vi "Load plugin from enum.vi"(4 "error in (no error)":errorcluster, 7 "Plugin type":T1) -> (0 "error out":errorcluster, 3 "Generic Plugin out":refnum<class "Generic Plugin.lvclass">)   [LabVIEW 2020, in "Generic Plugin.lvclass"]
uses:
  Generic Plugin.lvclass
  Plugin Type.ctl
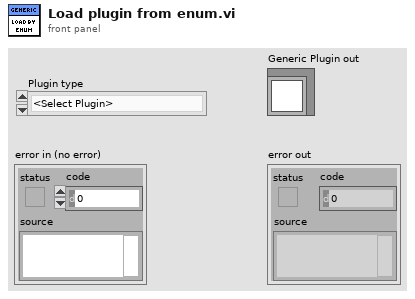
[diagram p1: front panel]
types:
  T1 = typedef "Generic Plugin.lvclass/Plugin Type.ctl" = enum16{"<Select Plugin>", "Orange", "Blue", "Red"}
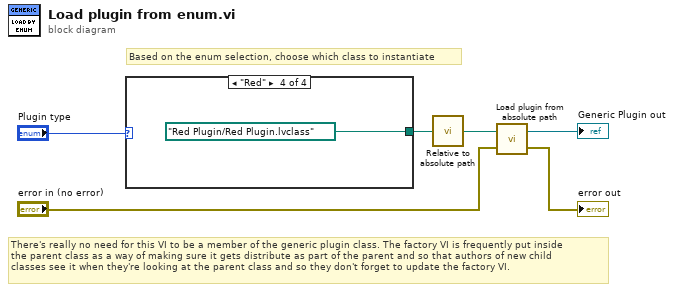
[diagram p0: block diagram]
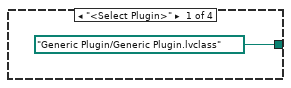
[diagram p2: hidden frame]
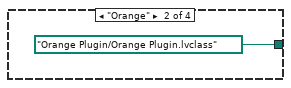
[diagram p3: hidden frame]
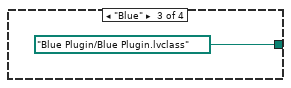
[diagram p4: hidden frame]
diagram:
  # "There's really no need for this VI to be a member of the generic plugin class. The factory VI is frequently put inside\nthe parent class as a way of making sure it gets distribute as part of the parent and so that authors of new child\nclasses see it when they're looking at the parent class and so they don't forget to update the factory VI."
  # "Based on the enum selection, choose which class to instantiate"
  n1 = case shown="\"Red\"" "Plugin type" {
    tunnel: [path "Generic Plugin/Generic Plugin.lvclass" path "Orange Plugin/Orange Plugin.lvclass" path "Blue Plugin/Blue Plugin.lvclass" path "Red Plugin/Red Plugin.lvclass"] -> w5
    frame "<Select Plugin>" {
    }
    frame "Orange" {
    }
    frame "Blue" {
    }
    frame "Red" {
    }
  }
  n2 = call "Relative to absolute path.vi"("Relative Path"=w5) -> ("Absolute Path"=w4:path)
  n3 = call "Load plugin from absolute path.vi"("error in (no error)"="error in (no error)", "Absolute Path"=w4) -> ("error out"=→"error out":errorcluster, "Generic Plugin out"=→"Generic Plugin out":refnum<class "Generic Plugin.lvclass">)
